vi "Untitled 2 (SubVI).vi"(8 "error in (no error)":errorcluster, 10 "direction":i32, 11 "VISA Refnum in":refnum<visa-resource-name>) -> (0 "error out":errorcluster, 1 "Slave":i32, 2 "Master":i32, 3 "VISA Refnum out":refnum<visa-resource-name>)   [LabVIEW 2011]
uses:
  <instrlib>/Newport ESP301/Newport ESP301.lvlib
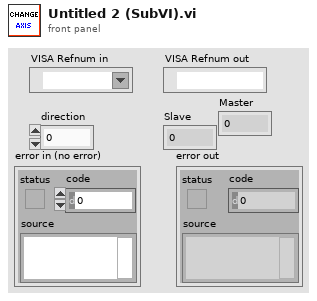
[diagram p1: front panel]
types:
  T1 = enum16{"Trapezoidal Mode", "S-curve Mode", "Jog Mode", "Slave to master's desired position (trajectory)", "Slave to master's actual position (feedback)", "Slave to master's actual velocity for jogging"}
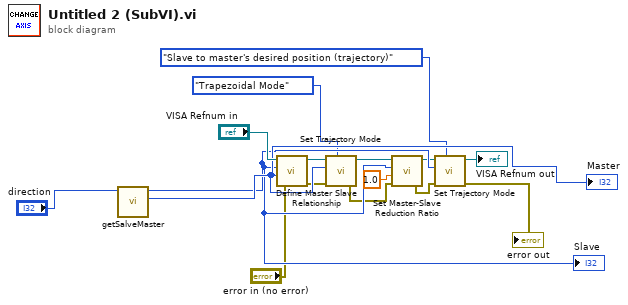
[diagram p0: block diagram]
diagram:
  n1 = call "getSalveMaster.vi"("direction in"="direction") -> ("Master"=w15:i32, "Slave"=w14:i32)  [unwired: 9 in]
  "Slave" <- w14
  "Master" <- w15
  n2 = call <instrlib>:"Define Master Slave Relationship.vi"("error in (no error)"="error in (no error)", "Master Axis"=w15, "Slave Axis"=w14, "VISA resource name"="VISA Refnum in") -> ("error out"=w5:errorcluster, "VISA resource name out"=w11:refnum<visa-resource-name>)  [unwired: 2 in]
  n3 = call <instrlib>:"Set Trajectory Mode.vi"("Trajectory Mode"=T1."Trapezoidal Mode", "error in (no error)"=w5, "Axis (1)"=w15, "VISA resource name"=w11) -> ("error out"=w4:errorcluster, "VISA resource name out"=w12:refnum<visa-resource-name>)  [unwired: 3 in]
  n4 = call <instrlib>:"Set Master-Slave Reduction Ratio.vi"("error in (no error)"=w4, "Reduction Ratio (0)"=1.0, "Axis (1)"=w14, "VISA resource name"=w12) -> ("error out"=w3:errorcluster, "VISA resource name out"=w13:refnum<visa-resource-name>)  [unwired: 2 in]
  n5 = call <instrlib>:"Set Trajectory Mode.vi"("Trajectory Mode"=T1."Slave to master's desired position (trajectory)", "error in (no error)"=w3, "Axis (1)"=w14, "VISA resource name"=w13) -> ("error out"=→"error out":errorcluster, "VISA resource name out"=→"VISA Refnum out":refnum<visa-resource-name>)  [unwired: 3 in]
